vi "Check Still Available.vi"(8 "error in (no error)":errorcluster, 11 "Output Actor Hardware in":refnum<class "Output Actor Hardware.lvclass">) -> (0 "error out":errorcluster, 3 "Output Actor Hardware out":refnum<class "Output Actor Hardware.lvclass">)   [LabVIEW 2015, in "Output Actor Hardware.lvclass"]
uses:
  Output Actor Hardware.lvclass
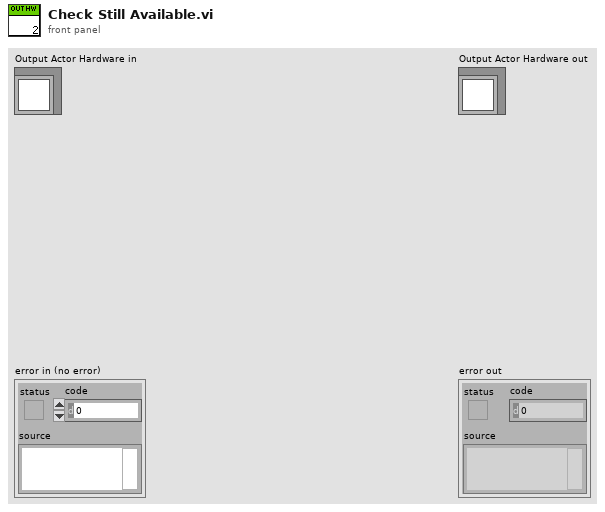
[diagram p1: front panel]
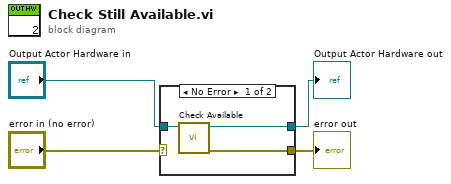
[diagram p0: block diagram]
diagram:
  n1 = case shown="No Error" "error in (no error)" {
    selector: "error in (no error)" -> [_ w9]
    tunnel: [w5 w9] -> w3
    tunnel: [w6 w8] -> w1
    tunnel: "Output Actor Hardware in" -> [w7 w8]
    frame No Error {
      n2 = call-dynamic "Check Available.vi"("Output Actor Hardware in"=w7) -> ("error out"=w5:errorcluster, "Output Actor Hardware out"=w6:refnum<class "Output Actor Hardware.lvclass">)  [unwired: 9 in]
    }
    frame Error {
    }
  }
  "error out" <- w3
  "Output Actor Hardware out" <- w1
